vi "Harmonic Distortion Analyzer.vi"   [LabVIEW 2020, in "NI_MAPro.lvlib"]
doc: "Takes a signal in and performs a full harmonic analysis, including measuring the fundamental frequency tone and harmonics, and returning the fundamental frequency, all harmonic amplitude levels, and the total harmonic distortion (THD). Wire data to the <B>signal in</B> input to determine the polymorphic instance to use or manually select the instance."
uses:
  NI_MAPro.lvlib
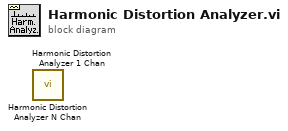
[diagram p0: block diagram]
diagram:
  n1 = call "Harmonic Distortion Analyzer N Chan.vi"() -> ()  [unwired: 6 in, 6 out]
  n2 = call "Harmonic Distortion Analyzer 1 Chan.vi"() -> ()  [unwired: 6 in, 6 out]
